vi "Layout Controls.vi"(7 "Control Cliuster In":refnum<vi>, 8 "Error In":errorcluster, 9 "NewBnds In":T2, 10 "Waveform Ref In":refnum<vi>, 11 "Controls Refs In":T1) -> (0 "Error Out":errorcluster)   [LabVIEW 2018, in "Waveform Control.xctl"]
doc: "Adjust the layout of the controls depending whether we are in wide or narrow mode"
uses:
  Waveform Control.xctl
  <vilib>/Utility/miscctls.llb/LVRectTypeDef.ctl
  <vilib>/Utility/miscctls.llb/LVPositionTypeDef.ctl
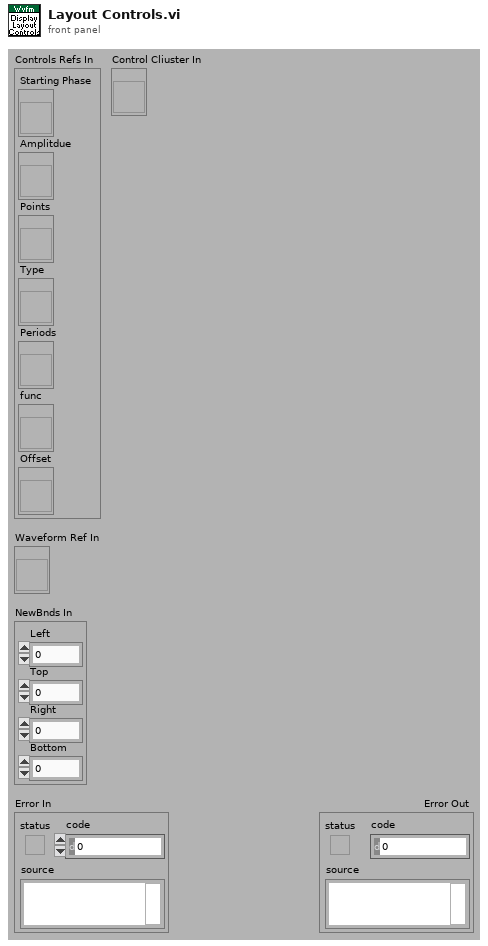
[diagram p1: front panel]
types:
  T1 = cluster{"Starting Phase":refnum<vi>, "Amplitdue":refnum<vi>, "Points":refnum<vi>, "Type":refnum<vi>, "Periods":refnum<vi>, "func":refnum<vi>, "Offset":refnum<vi>}
  T2 = typedef "LVRectTypeDef.ctl" = cluster{"Left":i16, "Top":i16, "Right":i16, "Bottom":i16}
  T3 = typedef "LVPositionTypeDef.ctl" = cluster{"Left":i32, "Top":i32}
  T4 = typedef "LVBoundsTypeDef.ctl" = cluster{"Width":u32, "Height":u32}
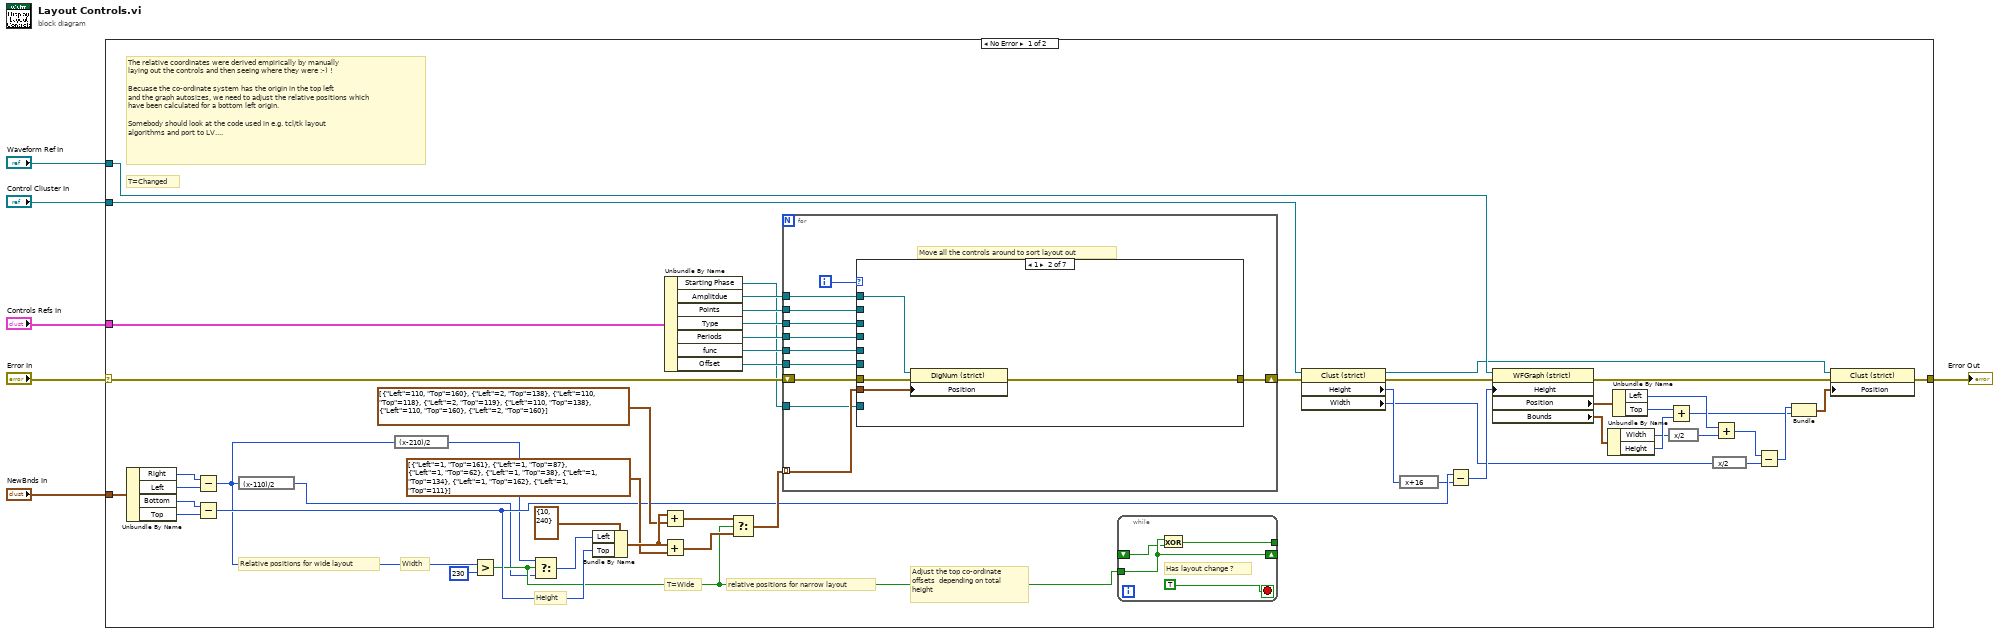
[diagram p0: block diagram]
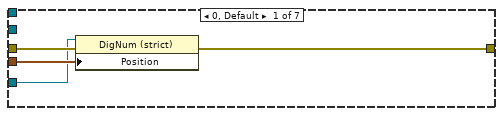
[diagram p2: hidden frame]
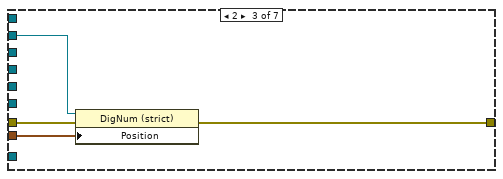
[diagram p3: hidden frame]
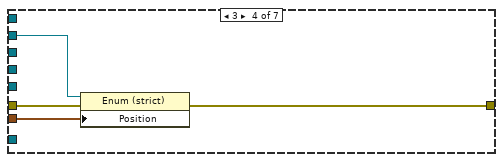
[diagram p4: hidden frame]
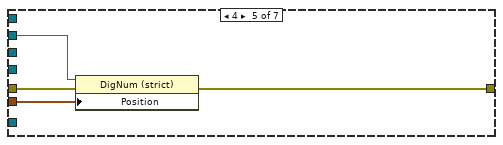
[diagram p5: hidden frame]
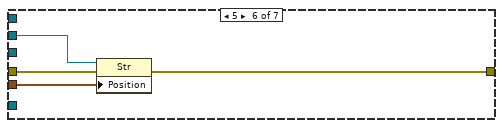
[diagram p6: hidden frame]
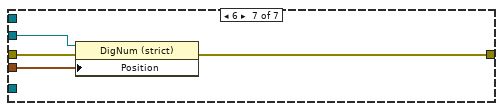
[diagram p7: hidden frame]
diagram:
  n1 = case shown="No Error" "Error In" {
    selector: "Error In" -> [w57 w101]
    tunnel: [w8 w101] -> w5
    tunnel: "NewBnds In" -> [w43 _]
    tunnel: "Waveform Ref In" -> [w42 _]
    tunnel: "Controls Refs In" -> [w41 _]
    tunnel: "Control Cliuster In" -> [w33 _]
    frame No Error {
      # "The relative coordinates were derived empirically by manually \nlaying out the controls and then seeing where they were :-) !\n\nBecuase the co-ordinate system has the origin in the top left\nand the graph autosizes, we need to adjust the relative positions which\nhave been calculated for a bottom left origin.\n\nSomebody should look at the code used in e.g. tcl/tk layout\nalgorithms and port to LV...."
      # "Adjust the top co-ordinate \noffsets  depending on total \nheight"
      # "T=Changed"
      # "relative positions for narrow layout"
      # "Relative positions for wide layout"
      # "T=Wide"
      # "Height"
      # "Width"
      n2 = Unbundle By Name(w43) -> ("Right"=w51:i16, "Left"=w53:i16, "Bottom"=w52:i16, "Top"=w54:i16)
      n3 = Subtract(x=w51, y=w53) -> (x-y=w24:i16)
      n4 = Subtract(x=w52, y=w54) -> (x-y=w31:i16)
      n5 = expression code="(x-110)/2"(w24) -> (w25:i16)
      n6 = expression code="(x-210)/2"(w24) -> (w26:i16)
      n7 = Greater?(x=w24, y=i16 230) -> (0:w27:bool)
      n8 = Select(t=w26, s=w27, f=w25) -> (s? t:f=w23:i16)
      n9 = Bundle By Name(cluster=T3 {"Left"=10, "Top"=240} ("Position"), "Left"=w23, "Top"=w31) -> (w55:T3)
      n10 = Add(x=w55, y=T3[] [{"Left"=110, "Top"=160}, {"Left"=2, "Top"=138}, {"Left"=110, "Top"=118}, {"Left"=2, "Top"=119}, {"Left"=110, "Top"=138}, {"Left"=110, "Top"=160}, {"Left"=2, "Top"=160}] ("appended array")) -> (x+y=w48:T3[])
      n11 = Add(x=w55, y=T3[] [{"Left"=1, "Top"=161}, {"Left"=1, "Top"=87}, {"Left"=1, "Top"=62}, {"Left"=1, "Top"=38}, {"Left"=1, "Top"=134}, {"Left"=1, "Top"=162}, {"Left"=1, "Top"=111}] ("appended array")) -> (x+y=w47:T3[])
      n12 = Unbundle By Name(w41) -> ("Starting Phase"=w34:refnum<vi>, "Amplitdue"=w40:refnum<vi>, "Points"=w39:refnum<vi>, "Type"=w38:refnum<vi>, "Periods"=w37:refnum<vi>, "func"=w36:refnum<vi>, "Offset"=w35:refnum<vi>)
      n13 = Select(t=w48, s=w27, f=w47) -> (s? t:f=w46:T3[])
      n14 = for {
        tunnel: w46 -> [w67] mode=indexing
        shift-right: [w66] -> w56
        shift-left: w57 -> [w65]
        tunnel: w34 -> [w64]
        tunnel: w40 -> [w63]
        tunnel: w39 -> [w62]
        tunnel: w38 -> [w61]
        tunnel: w37 -> [w60]
        tunnel: w36 -> [w59]
        tunnel: w35 -> [w58]
        i -> [w68]
        # "Move all the controls around to sort layout out"
        n15 = case shown="1" w68 {
          tunnel: w67 -> [w72 w76 w80 w84 w88 w92 w96]
          tunnel: [w71 w74 w78 w82 w86 w90 w94] -> w66
          tunnel: w65 -> [w70 w75 w79 w83 w87 w91 w95]
          tunnel: w64 -> [w69 _ _ _ _ _ _]
          tunnel: w63 -> [_ w73 _ _ _ _ _]
          tunnel: w62 -> [_ _ w77 _ _ _ _]
          tunnel: w61 -> [_ _ _ w81 _ _ _]
          tunnel: w60 -> [_ _ _ _ w85 _ _]
          tunnel: w59 -> [_ _ _ _ _ w89 _]
          tunnel: w58 -> [_ _ _ _ _ _ w93]
          frame 0, Default {
            n16 = property on="Property Node" class="DigNum (strict)"(reference=w69, error in=w70, "Position"=w72) -> (error out=w71:errorcluster)  [unwired: 1 out]
          }
          frame 1 {
            n17 = property on="Property Node" class="DigNum (strict)"(reference=w73, error in=w75, "Position"=w76) -> (error out=w74:errorcluster)  [unwired: 1 out]
          }
          frame 2 {
            n18 = property on="Property Node" class="DigNum (strict)"(reference=w77, error in=w79, "Position"=w80) -> (error out=w78:errorcluster)  [unwired: 1 out]
          }
          frame 3 {
            n19 = property on="Property Node" class="Enum (strict)"(reference=w81, error in=w83, "Position"=w84) -> (error out=w82:errorcluster)  [unwired: 1 out]
          }
          frame 4 {
            n20 = property on="Property Node" class="DigNum (strict)"(reference=w85, error in=w87, "Position"=w88) -> (error out=w86:errorcluster)  [unwired: 1 out]
          }
          frame 5 {
            n21 = property on="Property Node" class="Str"(reference=w89, error in=w91, "Position"=w92) -> (error out=w90:errorcluster)  [unwired: 1 out]
          }
          frame 6 {
            n22 = property on="Property Node" class="DigNum (strict)"(reference=w93, error in=w95, "Position"=w96) -> (error out=w94:errorcluster)  [unwired: 1 out]
          }
        }
      }
      n23 = while {
        shift-right: [w99] -> _
        shift-left: _ -> [w98]
        tunnel: w27 -> [w99]
        tunnel: [w97] -> _
        stop <- TRUE stop-if-true
        # "Has layout change ?"
        n24 = Exclusive Or(1:w98, 2:w99) -> (0:w97:bool)
      }
      n25 = property on="Property Node" class="Clust (strict)"(reference=w33, error in=w56) -> (reference out=w10:refnum<vi>, error out=w32:errorcluster, "Height"=w30:u32, "Width"=w14:u32)
      n26 = expression code="x+16"(w30) -> (w28:u32)
      n27 = Subtract(x=w31, y=w28) -> (x-y=w29:u32)
      n28 = property on="Property Node" class="WFGraph (strict)"(reference=w42, error in=w32, "Height"=w29) -> (error out=w9:errorcluster, "Position"=w22:T3, "Bounds"=w21:T4)  [unwired: 1 out]
      n29 = Unbundle By Name(w21) -> ("Width"=w17:u32, "Height"=w19:u32)
      n30 = Unbundle By Name(w22) -> ("Left"=w18:i32, "Top"=w20:i32)
      n31 = Add(x=w20, y=w19) -> (x+y=w11:u32)
      n32 = expression code="x/2"(w17) -> (w16:u32)
      n33 = expression code="x/2"(w14) -> (w13:u32)
      n34 = Add(x=w18, y=w16) -> (x+y=w15:u32)
      n35 = Subtract(x=w15, y=w13) -> (x-y=w12:u32)
      n36 = Bundle(w12, w11) -> (w7:cluster{u32, u32})  [unwired: 1 out]
      n37 = property class="Clust (strict)"(reference=w10, error in=w9, "Position"=w7) -> (error out=w8:errorcluster)  [unwired: 1 out]
    }
    frame Error {
    }
  }
  "Error Out" <- w5
